vi "LV_multiports_multiservers_2.vi"() -> ()   [LabVIEW 2020]
panel:
  in  "Send Test Img":bool
  in  "h":i32=10 min=1 max=5000 step=1
  in  "w":i32=1 min=1 max=5000 step=1
  out "Elaps ms":u32
  in  "Send Image":bool
  out "Path to Python script":path
  in  "Stop":bool
  out "Answer":string
  in  "Ping":bool
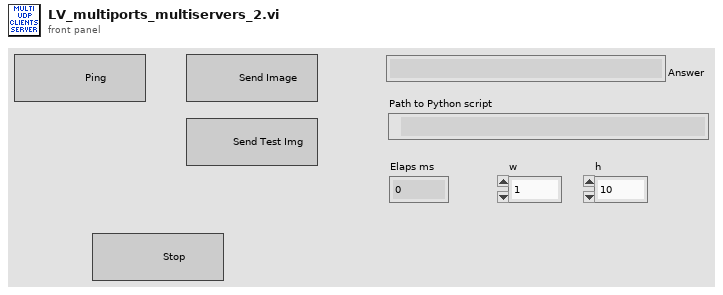
[diagram p1: front panel]
types:
  T1 = enum8{"Enabled", "Disabled", "Disabled and Grayed Out"}
  T2 = typedef "Image Type" = u32
  T3 = typedef "IMAQ Image.ctl" = refnum<image>
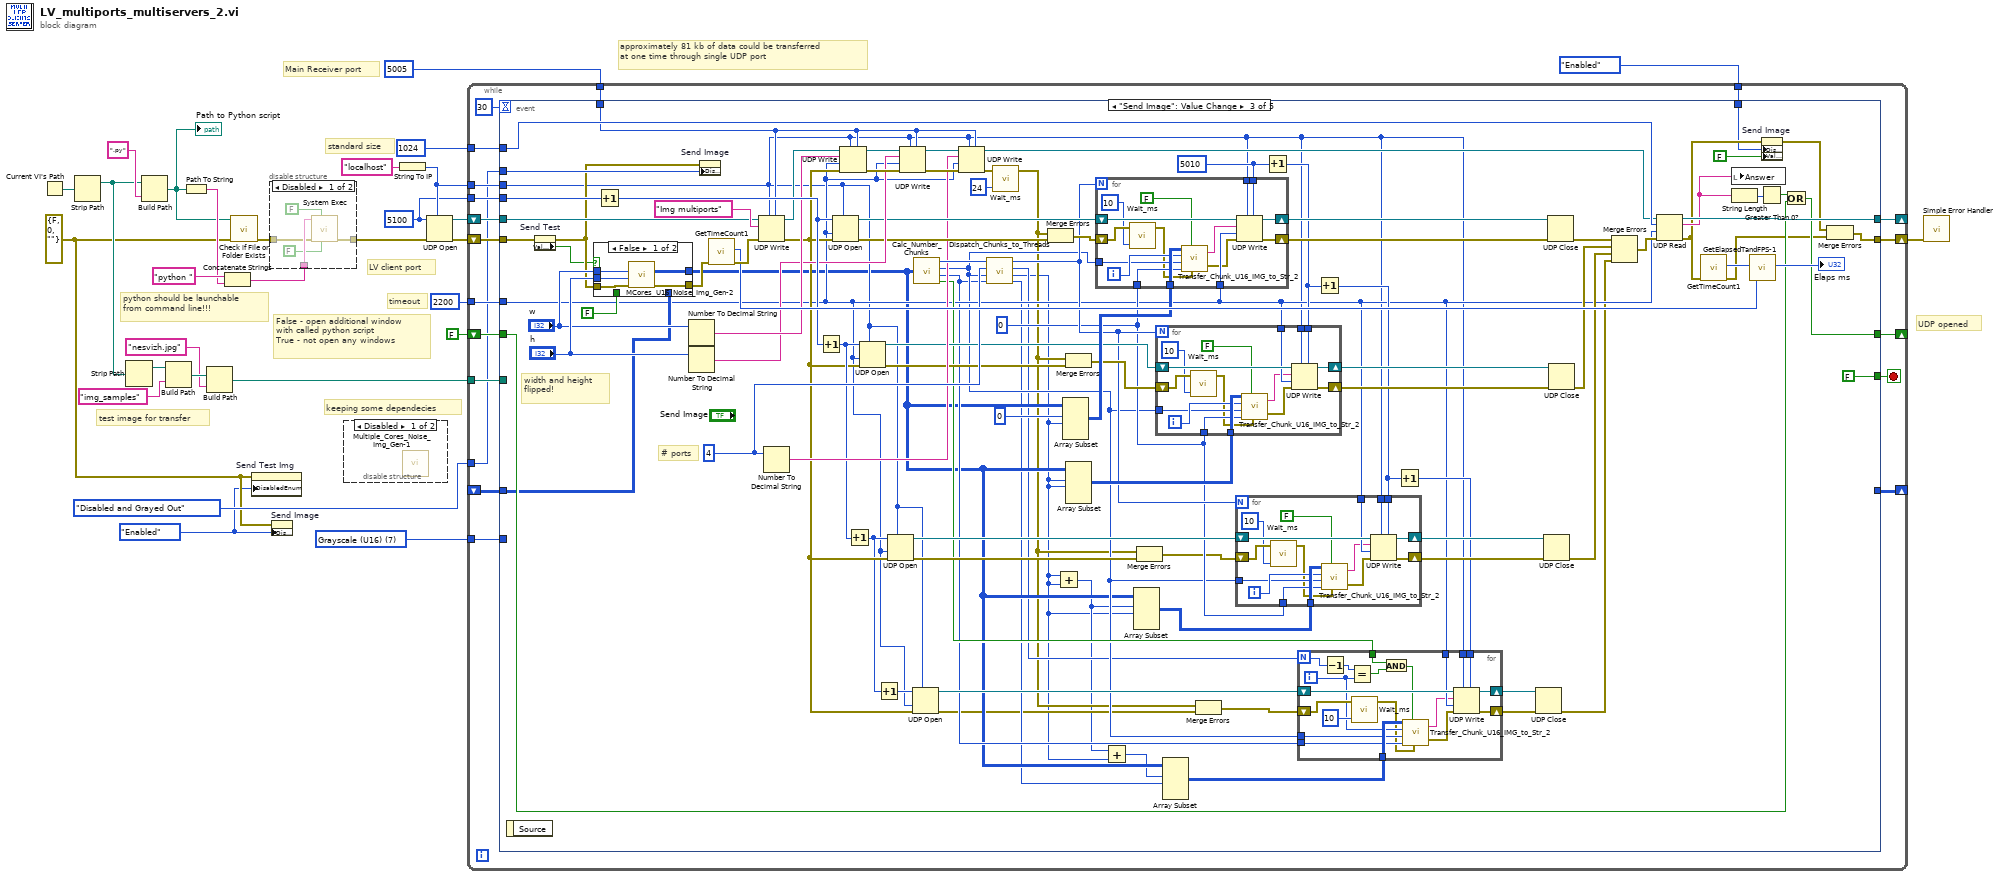
[diagram p0: block diagram]
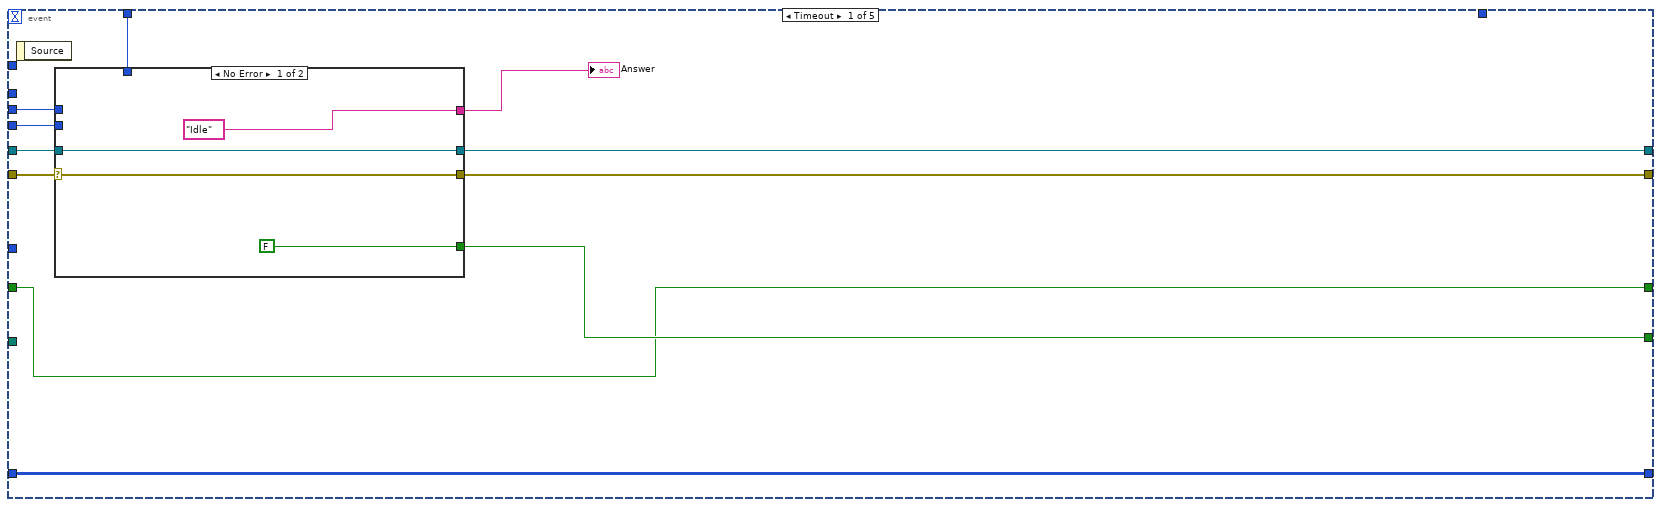
[diagram p4: hidden frame]
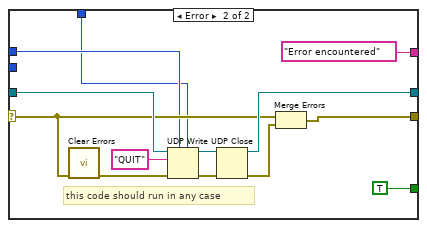
[diagram p5: hidden frame]
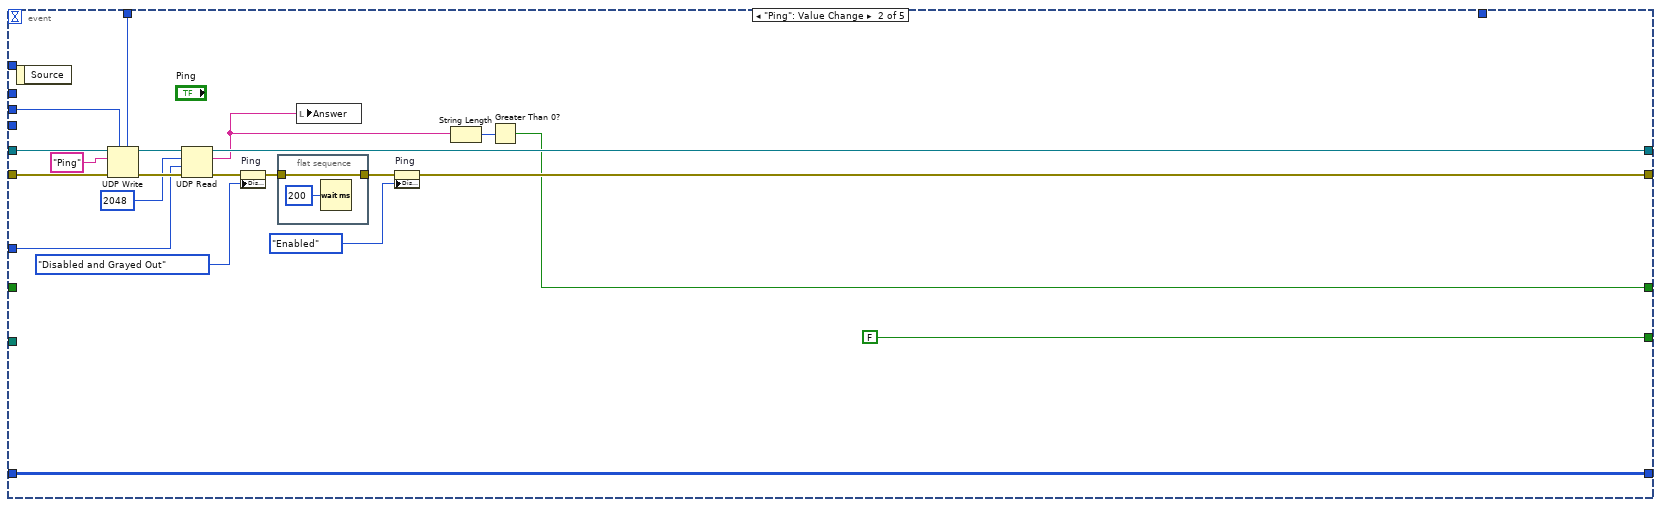
[diagram p6: hidden frame]
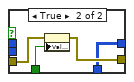
[diagram p7: hidden frame]
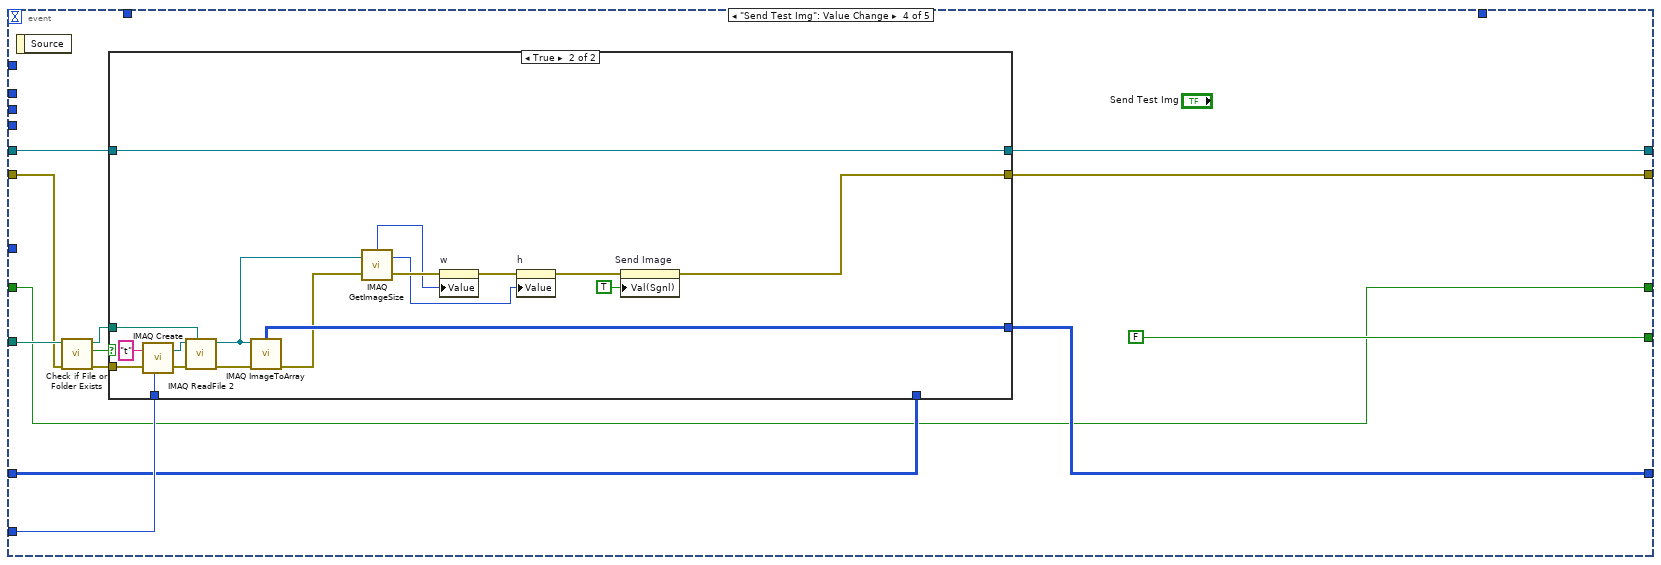
[diagram p8: hidden frame]
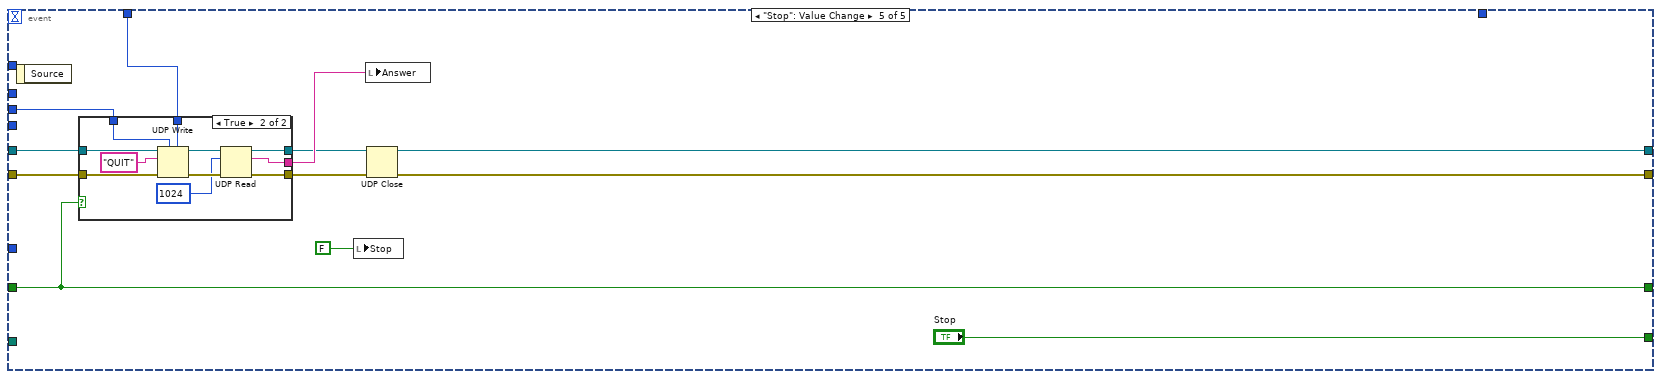
[diagram p10: hidden frame]
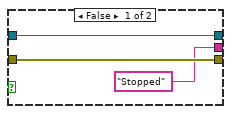
[diagram p11: hidden frame]
diagram:
  w1 = T1."Enabled" ("Disabled")
  w7 = T2 7 items=["Grayscale (U8)", "Grayscale (I16)", "Grayscale (SGL)", "Complex (CSG)", "RGB (U32)", "HSL (U32)", "RGB (U64)", "Grayscale (U16)"] ("Image Type")
  w16 = u16 5100 ("remote port or service name")
  w2 = errorcluster {"status"=FALSE, "code"=0, "source"=""} ("error in (no error)")
  # "approximately 81 kb of data could be transferred \nat one time through single UDP port"
  # "standard size"
  # "UDP opened"
  # "test image for transfer"
  # "keeping some dependecies"
  # "timeout"
  # "Main Receiver port"
  # "LV client port"
  # "False - open additional window\nwith called python script\nTrue - not open any windows"
  # "python should be launchable \nfrom command line!!!"
  n1 = Current VI's Path() -> (path=w28:path)
  n2 = Strip Path(path=w28) -> (stripped path=w13:path)  [unwired: 1 out]
  n3 = Strip Path(path=w13) -> (stripped path=w12:path)  [unwired: 1 out]
  n4 = Build Path(base path=w13, name or relative path=".py" ("string")) -> (appended path=w23:path)
  "Path to Python script" <- w23
  n5 = Build Path(base path=w12, name or relative path="img_samples" ("string")) -> (appended path=w10:path)
  n6 = Path To String(path=w23) -> (string=w24:string)
  n7 = Build Path(base path=w10, name or relative path="nesvizh.jpg" ("string")) -> (appended path=w8:path)
  n8 = Concatenate Strings("python " ("command line"), w24) -> (w26:string)
  n9 = call <vilib>:"Check if File or Folder Exists.vi"("error in (no error)"=w2, "path"=w23) -> ("error out"=w22:errorcluster)  [unwired: 7 in, 2 out]
  n10 = property on="Send Test Img" class="Bool (strict)"(error in=w2, "DisabledEnum"=w1) -> ()  [unwired: 1 in, 2 out]
  n11 = disable-structure shown="Disabled" {
    disable-tunnel: w26 -> [w34 _]
    disable-tunnel: [w33 w35] -> w21
    disable-tunnel: w22 -> [w31 w35]
    frame Disabled {
      n12 = call <vilib>:"System Exec.vi"("run minimized? (F)"=FALSE, "wait until completion? (T)"=FALSE, "error in (no error)"=w31, "command line"=w34) -> ("error out"=w33:errorcluster)  [unwired: 4 in, 3 out]
    }
    frame Enabled {
    }
  }
  n13 = property on="Send Image" class="Bool (strict)"(error in=w2, "DisabledEnum"=w1) -> ()  [unwired: 1 in, 2 out]
  n14 = disable-structure shown="Disabled" {
    frame Disabled {
      n15 = call "Multiple_Cores_Noise_Img_Gen-1.vi"() -> ()  [unwired: 10 in, 2 out]
    }
    frame Enabled {
    }
  }
  n16 = String To IP(1:"localhost" ("address")) -> (0:w17:u32)
  n17 = UDP Open(7:w17, 8:w21, 11:w16) -> (port=w19:refnum<k16>, 0:w20:errorcluster)  [unwired: 2 in, 1 out]
  n18 = while {
    shift-right: [w51] -> _
    shift-left: w19 -> [w52]
    shift-right: [w49] -> w29
    shift-left: w20 -> [w53]
    tunnel: w17 -> [w47]
    tunnel: w16 -> [w48]
    tunnel: u16 5005 ("remote port or service name") -> [w46]
    tunnel: 2200 -> [w45]
    tunnel: w8 -> [w44]
    tunnel: w7 -> [w43]
    shift-right: [w41] -> _
    shift-left: FALSE -> [w42]
    tunnel: 1024 -> [w40]
    tunnel: T1."Disabled and Grayed Out" ("Disabled") -> [w39]
    tunnel: T1."Enabled" ("Disabled") -> [w38]
    shift-right: [w37] -> _
    shift-left: _ -> [w36]
    stop <- w50 stop-if-true
    n19 = event shown="[2] \"Send Image\": Value Change" {
      selector: _ -> [_ _ _ _ _]
      dyn-events: _ -> [_ _ _ _ _]
      timeout: 30 -> [_ _ _ _ _]
      tunnel: [w61 FALSE ("Stop") FALSE ("Stop") FALSE ("Stop") "Stop"] -> w50
      tunnel: w53 -> [w65 w97 w150 w290 w320]
      tunnel: w52 -> [w64 w96 w201 w285 w321]
      tunnel: [w63 w92 w199 w283 w322] -> w51
      tunnel: [w62 w99 w153 w284 w323] -> w49
      tunnel: w48 -> [w59 _ w189 _ _]
      tunnel: w47 -> [w58 w89 w121 _ w316]
      tunnel: w46 -> [w57 w88 w175 _ w315]
      tunnel: w45 -> [_ w87 w122 _ _]
      tunnel: w44 -> [_ _ _ w291 _]
      tunnel: w43 -> [_ _ _ w286 _]
      tunnel: w42 -> [w56 _ w191 w280 w314]
      tunnel: [w56 w84 w190 w280 w314] -> w41
      tunnel: w40 -> [_ _ w188 _ _]
      tunnel: w39 -> [_ _ w157 _ _]
      tunnel: w38 -> [_ _ w155 _ _]
      tunnel: [w55 w83 _ w282 _] -> w37
      tunnel: w36 -> [w55 w83 w146 w281 _]
      event Timeout {
        n20 = event-data() -> ()  [unwired: 1 in, 1 out]
        n21 = case shown="No Error" w65 {
          selector: w65 -> [w68 w77]
          tunnel: [w69 w80] -> w63
          tunnel: w64 -> [w69 w79]
          tunnel: [w68 w78] -> w62
          tunnel: [FALSE ("Stop") TRUE ("Stop")] -> w61
          tunnel: ["Idle" ("Answer") "Error encountered" ("Answer")] -> w60
          tunnel: w59 -> [_ _]
          tunnel: w58 -> [_ w76]
          tunnel: w57 -> [_ w75]
          frame No Error {
          }
          frame Error {
            # "this code should run in any case"
            n22 = call <vilib>:"Clear Errors.vi"("error in (no error)"=w77) -> ("error out"=w74:errorcluster)  [unwired: 5 in, 1 out]
            n23 = UDP Write(address=w76, port or service name=w75, connection ID=w79, data in="QUIT", 8:w74) -> (error out=w73:errorcluster, 3:w71:refnum<k16>)  [unwired: 1 in]
            n24 = UDP Close(connection ID=w71, 8:w73) -> (connection ID out=w80:refnum<k16>, error out=w70:errorcluster)
            n25 = Merge Errors(w77, w70) -> (w78:errorcluster)
          }
        }
        "Answer" <- w60
      }
      event "Ping": Value Change {
        n26 = event-data() -> ()  [unwired: 1 in, 1 out]
        n27 = UDP Write(address=w89, port or service name=w88, connection ID=w96, data in="Ping", 8:w97) -> (error out=w94:errorcluster, 3:w93:refnum<k16>)  [unwired: 1 in]
        n28 = UDP Read(connection ID=w93, max size (548)=2048 ("bytes to read"), timeout ms (25000)=w87, 8:w94) -> (data out=w86:string, error out=w91:errorcluster, 3:w92:refnum<k16>)  [unwired: 2 out]
        n29 = property on="Ping" class="Bool"(error in=w91, "DisabledEnum"=T1."Disabled and Grayed Out" ("Disabled")) -> (error out=w102:errorcluster)  [unwired: 1 in, 1 out]
        n30 = flat-sequence {
          tunnel: w102 -> [w104]
          tunnel: [w104] -> w100
          frame #0 {
            n31 = Wait (ms)(milliseconds to wait=u32 200) -> ()  [unwired: 1 out]
          }
        }
        n32 = local write "Answer"(w86) -> ()
        n33 = property on="Ping" class="Bool"(error in=w100, "DisabledEnum"=T1."Enabled" ("Disabled")) -> (error out=w99:errorcluster)  [unwired: 1 in, 1 out]
        n34 = String Length(string=w86) -> (length=w85:i32)
        n35 = Greater Than 0?(x=w85) -> (x > 0?=w84:bool)
      }
      event "Send Image": Value Change {
        w136 = 0 ("[IN] # rows last transfer")
        w164 = u16 5010 ("remote port or service name")
        w165 = 4
        # "# ports"
        # "width and height \nflipped!"
        n36 = event-data() -> ()  [unwired: 1 in, 1 out]
        n37 = property on="Send Test" class="Bool (strict)"(error in=w150) -> (error out=w149:errorcluster, "Value"=w148:bool)  [unwired: 1 in, 1 out]
        n38 = case shown="False" w148 {
          tunnel: "h" -> [w259 _]
          tunnel: "w" -> [w258 _]
          tunnel: [w257 w261] -> w158
          tunnel: w149 -> [w256 w263]
          tunnel: [w255 w260] -> w115
          tunnel: FALSE ("Send Test Img") -> [_ w262]
          tunnel: w146 -> [_ w260]
          frame False {
            n39 = call "MCores_U16_Noise_Img_Gen-2.vi"("error IN"=w256, "[IN] Width"=w259, "[IN] Height"=w258) -> ("error OUT"=w257:errorcluster, "[OUT] U16 Pixel Img"=w255:u16[][])  [unwired: 7 in]
          }
          frame True {
            n40 = property on="Send Test Img" class="Bool (strict)"(error in=w263, "Value"=w262) -> (error out=w261:errorcluster)  [unwired: 1 in, 1 out]
          }
        }
        n41 = Increment(x=w189) -> (x+1=w187:u16)
        n42 = Number To Decimal String(number="w") -> (decimal integer string=w185:string)  [unwired: 1 in]
        n43 = Number To Decimal String(number="h") -> (decimal integer string=w182:string)  [unwired: 1 in]
        n44 = property on="Send Image" class="Bool (strict)"(error in=w149, "DisabledEnum"=w157) -> ()  [unwired: 1 in, 2 out]
        n45 = call "GetTimeCount1.vi"("error IN"=w158) -> ("error OUT"=w198:errorcluster, "[OUT] Timer Count"=w196:u32)  [unwired: 9 in]
        n46 = UDP Write(address=w121, port or service name=w175, connection ID=w201, data in="Img multiports", 8:w198) -> (error out=w129:errorcluster, 3:w186:refnum<k16>)  [unwired: 1 in]
        n47 = Number To Decimal String(number=w165) -> (decimal integer string=w163:string)  [unwired: 1 in]
        n48 = Increment(x=w187) -> (x+1=w145:u16)
        n49 = UDP Open(7:w121, 8:w129, 9:w122, 11:w187) -> (port=w172:refnum<k16>, 0:w167:errorcluster)  [unwired: 1 in, 1 out]
        n50 = UDP Write(address=w121, port or service name=w175, connection ID=w186, data in=w185, 8:w129, 9:w122) -> (error out=w184:errorcluster, 3:w183:refnum<k16>)
        n51 = Increment(x=w145) -> (x+1=w128:u16)
        n52 = UDP Open(7:w121, 8:w129, 9:w122, 11:w145) -> (port=w143:refnum<k16>, 0:w162:errorcluster)  [unwired: 1 in, 1 out]
        n53 = Increment(x=w128) -> (x+1=w127:u16)
        n54 = UDP Open(7:w121, 8:w129, 9:w122, 11:w128) -> (port=w137:refnum<k16>, 0:w135:errorcluster)  [unwired: 1 in, 1 out]
        n55 = UDP Write(address=w121, port or service name=w175, connection ID=w183, data in=w182, 8:w184, 9:w122) -> (error out=w177:errorcluster, 3:w176:refnum<k16>)
        n56 = UDP Open(7:w121, 8:w129, 9:w122, 11:w127) -> (port=w126:refnum<k16>, 0:w111:errorcluster)  [unwired: 1 in, 1 out]
        n57 = call "Calc_Number_Chunks.vi"("[IN] U16 Pixel Img"=w115) -> ("[OUT] Number of chunks"=w178:i32, "[OUT] # rows single transfer"=w120:i32, "[OUT] # rows last transfer"=w119:i32, "[OUT] Not-equal last transfer"=w125:bool)
        n58 = UDP Write(address=w121, port or service name=w175, connection ID=w176, data in=w163, 8:w177, 9:w122) -> (error out=w168:errorcluster, 3:w174:refnum<k16>)
        n59 = call "Dispatch_Chunks_to_Threads.vi"("[IN] # rows last transfer"=w119, "[IN] # rows single transfer"=w120, "[IN] Number of threads"=w165, "[IN] Number of chunks"=w178) -> ("[OUT] Remained rows last transfer"=w113:i32, "[OUT] Rows of img for port"=w107:i32, "[OUT] Dispatched lastly"=w114:i32, "[OUT] Dispatched chunks"=w139:i32)
        n60 = call "Wait_ms.vi"("[IN] Suspend ms"=u32 24, "error IN"=w168) -> ("error OUT"=w112:errorcluster)  [unwired: 3 in]
        n61 = Merge Errors(w112, w167) -> (w166:errorcluster)
        n62 = Add(x=w107, y=w107) -> (x+y=w108:i32)
        n63 = Array Subset(array=w115, index (row)=0 ("index"), length (row)=w107) -> (w161:u16[][])  [unwired: 2 in]
        n64 = Merge Errors(w112, w162) -> (w144:errorcluster)
        n65 = Array Subset(array=w115, index (row)=w107, length (row)=w107) -> (w140:u16[][])  [unwired: 2 in]
        n66 = for {
          N: w139 -> [_]
          shift-right: [w279] -> w170
          shift-left: w166 -> [w273]
          shift-right: [w278] -> w171
          shift-left: w172 -> [w277]
          tunnel: w121 -> [w276]
          tunnel: w164 -> [w275]
          tunnel: w120 -> [w266]
          tunnel: w161 -> [w268]
          tunnel: w122 -> [w274]
          tunnel: w136 -> [w265]
          i -> [w267]
          n67 = call "Wait_ms.vi"("[IN] Suspend ms"=u32 10, "error IN"=w273) -> ("error OUT"=w264:errorcluster)  [unwired: 3 in]
          n68 = call "Transfer_Chunk_U16_IMG_to_Str_2.vi"("error IN"=w264, "[IN] Use remained rows"=FALSE, "[IN] # rows last transfer"=w265, "[IN] # rows single transfer"=w266, "[IN] # of chunk"=w267, "[IN] U16 Pixel Img"=w268) -> ("error OUT"=w269:errorcluster, "[OUT] Converted String"=w270:string)
          n69 = UDP Write(address=w276, port or service name=w275, connection ID=w277, data in=w270, 8:w269, 9:w274) -> (error out=w279:errorcluster, 3:w278:refnum<k16>)
        }
        n70 = Add(x=w108, y=w107) -> (x+y=w106:i32)
        n71 = Array Subset(array=w115, index (row)=w108, length (row)=w107) -> (w130:u16[][])  [unwired: 2 in]
        n72 = Merge Errors(w112, w135) -> (w134:errorcluster)
        n73 = Array Subset(array=w115, index (row)=w106, length (row)=w113) -> (w109:u16[][])  [unwired: 2 in]
        n74 = Merge Errors(w112, w111) -> (w110:errorcluster)
        n75 = Increment(x=w164) -> (x+1=w138:u16)
        n76 = for {
          N: w139 -> [_]
          shift-right: [w254] -> w141
          shift-left: w144 -> [w248]
          shift-right: [w253] -> w142
          shift-left: w143 -> [w252]
          tunnel: w121 -> [w251]
          tunnel: w138 -> [w250]
          tunnel: w120 -> [w241]
          tunnel: w140 -> [w243]
          tunnel: w122 -> [w249]
          tunnel: w136 -> [w240]
          i -> [w242]
          n77 = call "Wait_ms.vi"("[IN] Suspend ms"=u32 10, "error IN"=w248) -> ("error OUT"=w239:errorcluster)  [unwired: 3 in]
          n78 = call "Transfer_Chunk_U16_IMG_to_Str_2.vi"("error IN"=w239, "[IN] Use remained rows"=FALSE, "[IN] # rows last transfer"=w240, "[IN] # rows single transfer"=w241, "[IN] # of chunk"=w242, "[IN] U16 Pixel Img"=w243) -> ("error OUT"=w244:errorcluster, "[OUT] Converted String"=w245:string)
          n79 = UDP Write(address=w251, port or service name=w250, connection ID=w252, data in=w245, 8:w244, 9:w249) -> (error out=w254:errorcluster, 3:w253:refnum<k16>)
        }
        n80 = Increment(x=w138) -> (x+1=w124:u16)
        n81 = for {
          N: w139 -> [_]
          shift-right: [w238] -> w132
          shift-left: w134 -> [w232]
          shift-right: [w237] -> w133
          shift-left: w137 -> [w236]
          tunnel: w121 -> [w235]
          tunnel: w124 -> [w234]
          tunnel: w120 -> [w225]
          tunnel: w130 -> [w227]
          tunnel: w122 -> [w233]
          tunnel: w136 -> [w224]
          i -> [w226]
          n82 = call "Wait_ms.vi"("[IN] Suspend ms"=u32 10, "error IN"=w232) -> ("error OUT"=w223:errorcluster)  [unwired: 3 in]
          n83 = call "Transfer_Chunk_U16_IMG_to_Str_2.vi"("error IN"=w223, "[IN] Use remained rows"=FALSE, "[IN] # rows last transfer"=w224, "[IN] # rows single transfer"=w225, "[IN] # of chunk"=w226, "[IN] U16 Pixel Img"=w227) -> ("error OUT"=w228:errorcluster, "[OUT] Converted String"=w229:string)
          n84 = UDP Write(address=w235, port or service name=w234, connection ID=w236, data in=w229, 8:w228, 9:w233) -> (error out=w238:errorcluster, 3:w237:refnum<k16>)
        }
        n85 = Increment(x=w124) -> (x+1=w123:u16)
        n86 = for {
          N: w114 -> [w222]
          shift-right: [w218] -> w117
          shift-left: w110 -> [w212]
          tunnel: w109 -> [w209]
          tunnel: w120 -> [w207]
          tunnel: w119 -> [w206]
          shift-right: [w217] -> w118
          shift-left: w126 -> [w216]
          tunnel: w125 -> [w220]
          tunnel: w121 -> [w215]
          tunnel: w123 -> [w214]
          tunnel: w122 -> [w213]
          i -> [w208]
          n87 = Decrement(x=w222) -> (x-1=w221:i32)
          n88 = Equal?(x=w221, y=w208) -> (x = y?=w219:bool)
          n89 = call "Wait_ms.vi"("[IN] Suspend ms"=u32 10, "error IN"=w212) -> ("error OUT"=w205:errorcluster)  [unwired: 3 in]
          n90 = And(x=w220, y=w219) -> (x .and. y?=w210:bool)
          n91 = call "Transfer_Chunk_U16_IMG_to_Str_2.vi"("error IN"=w205, "[IN] Use remained rows"=w210, "[IN] # rows last transfer"=w206, "[IN] # rows single transfer"=w207, "[IN] # of chunk"=w208, "[IN] U16 Pixel Img"=w209) -> ("error OUT"=w203:errorcluster, "[OUT] Converted String"=w204:string)
          n92 = UDP Write(address=w215, port or service name=w214, connection ID=w216, data in=w204, 8:w203, 9:w213) -> (error out=w218:errorcluster, 3:w217:refnum<k16>)
        }
        n93 = UDP Close(connection ID=w118, 8:w117) -> (error out=w116:errorcluster)  [unwired: 1 out]
        n94 = UDP Close(connection ID=w133, 8:w132) -> (error out=w131:errorcluster)  [unwired: 1 out]
        n95 = UDP Close(connection ID=w171, 8:w170) -> (error out=w181:errorcluster)  [unwired: 1 out]
        n96 = UDP Close(connection ID=w142, 8:w141) -> (error out=w179:errorcluster)  [unwired: 1 out]
        n97 = Merge Errors(w181, w179, w131, w116) -> (w180:errorcluster)
        n98 = UDP Read(connection ID=w174, max size (548)=w188, timeout ms (25000)=w122, 8:w180) -> (data out=w193:string, error out=w156:errorcluster, 3:w199:refnum<k16>)  [unwired: 2 out]
        n99 = call "GetTimeCount1.vi"("error IN"=w156) -> ("error OUT"=w152:errorcluster, "[OUT] Timer Count"=w197:u32)  [unwired: 9 in]
        n100 = local write "Answer"(w193) -> ()
        n101 = String Length(string=w193) -> (length=w194:i32)
        n102 = call "GetElapsedTandFPS-1.vi"("[IN] Timer Count Before ALL [ms]"=w196, "[IN] Timer Count After ALL [ms]"=w197) -> ("[OUT] Elapsed time [ms]"=→"Elaps ms":u32)  [unwired: 3 in, 2 out]
        n103 = Greater Than 0?(x=w194) -> (x > 0?=w192:bool)
        n104 = property on="Send Image" class="Bool (strict)"(error in=w156, "DisabledEnum"=w155, "Value"=FALSE ("Send Image")) -> (error out=w154:errorcluster)  [unwired: 1 in, 1 out]
        n105 = Or(x=w192, y=w191) -> (x .or. y?=w190:bool)
        n106 = Merge Errors(w154, w152) -> (w153:errorcluster)
      }
      event "Send Test Img": Value Change {
        n107 = event-data() -> ()  [unwired: 1 in, 1 out]
        n108 = call <vilib>:"Check if File or Folder Exists.vi"("error in (no error)"=w290, "path"=w291) -> ("error out"=w289:errorcluster, "file or folder exists?"=w288:bool, "dup path"=w287:path)  [unwired: 7 in]
        n109 = case shown="True" w288 {
          tunnel: w289 -> [w294 w313]
          tunnel: w287 -> [_ w308]
          tunnel: w286 -> [_ w312]
          tunnel: w285 -> [w295 w300]
          tunnel: [w294 w298] -> w284
          tunnel: [w295 w300] -> w283
          tunnel: [w293 w303] -> w282
          tunnel: w281 -> [w293 _]
          frame False {
          }
          frame True {
            n110 = call "IMAQ Create"("Image Name"="t", "Image Type"=w312, "error in (no error)"=w313) -> ("New Image"=w309:T3, "error out"=w310:errorcluster)  [unwired: 2 in]
            n111 = call "IMAQ ReadFile 2"("File Path"=w308, "error in (no error)"=w310, "Image"=w309) -> ("error out"=w306:errorcluster, "Image Out"=w307:T3)  [unwired: 4 in, 3 out]
            n112 = call "IMAQ ImageToArray"("error in (no error)"=w306, "Image"=w307) -> ("error out"=w302:errorcluster, "Image Pixels (U8)"=w303:u8[][])  [unwired: 2 in, 3 out]
            n113 = call "IMAQ GetImageSize"("Image"=w307, "error in (no error)"=w302) -> ("Y Resolution"=w296:i32, "X Resolution"=w297:i32, "error out"=w305:errorcluster)  [unwired: 2 in]
            n114 = property on="w" class="DigNum (strict)"(error in=w305, "Value"=w297) -> (error out=w304:errorcluster)  [unwired: 1 in, 1 out]
            n115 = property on="h" class="DigNum (strict)"(error in=w304, "Value"=w296) -> (error out=w301:errorcluster)  [unwired: 1 in, 1 out]
            n116 = property on="Send Image" class="Bool (strict)"(error in=w301, "Val(Sgnl)"=TRUE ("Value (Signaling)")) -> (error out=w298:errorcluster)  [unwired: 1 in, 1 out]
          }
        }
      }
      event "Stop": Value Change {
        n117 = event-data() -> ()  [unwired: 1 in, 1 out]
        n118 = case shown="True" w314 {
          tunnel: w321 -> [w328 w339]
          tunnel: w320 -> [w327 w338]
          tunnel: [w327 w334] -> w319
          tunnel: ["Stopped" ("data out") w333] -> w318
          tunnel: [w328 w332] -> w317
          tunnel: w316 -> [_ w330]
          tunnel: w315 -> [_ w329]
          frame False {
          }
          frame True {
            n119 = UDP Write(address=w330, port or service name=w329, connection ID=w339, data in="QUIT", 8:w338) -> (error out=w335:errorcluster, 3:w336:refnum<k16>)  [unwired: 1 in]
            n120 = UDP Read(connection ID=w336, max size (548)=1024 ("bytes to read"), 8:w335) -> (data out=w333:string, error out=w334:errorcluster, 3:w332:refnum<k16>)  [unwired: 1 in, 2 out]
          }
        }
        n121 = local write "Stop"(FALSE ("Stop")) -> ()
        n122 = local write "Answer"(w318) -> ()
        n123 = UDP Close(connection ID=w317, 8:w319) -> (connection ID out=w322:refnum<k16>, error out=w323:errorcluster)
      }
    }
  }
  n124 = call <vilib>:"Simple Error Handler.vi"("error in (no error)"=w29) -> ()  [unwired: 4 in, 5 out]
